vi "ZPL CheckSum Append.vi"(8 "error":errorcluster, 10 "Input Cmd":string, 11 "VISA":refnum<visa-resource-name>="COM1") -> (0 "error out":errorcluster, 2 "ChkSum Cmd":string, 3 "VISA out":refnum<visa-resource-name>)   [LabVIEW 2016]
doc: "This vi will add a checksum to any command string.\nThe format of the \"ChkSum Cmd\" output is:\n \"Command\" & \"Dollar Sign\" & \"Two Hex Digits\" & \"Carriage Return\"\n\nThe command is only formulated, it is not sent to the instrument."
panel:
  # "Add Checksum to \n  Command"
  # "Lambda ZPLUS \n  DC Power Supplies"
  # "Append \"$xx\" checksum to any\ncommand string if it is not already done"
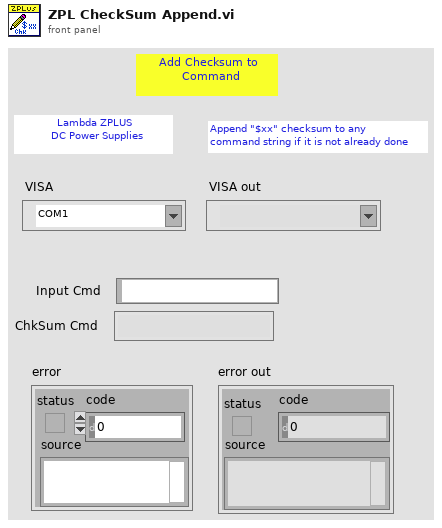
[diagram p1: front panel]
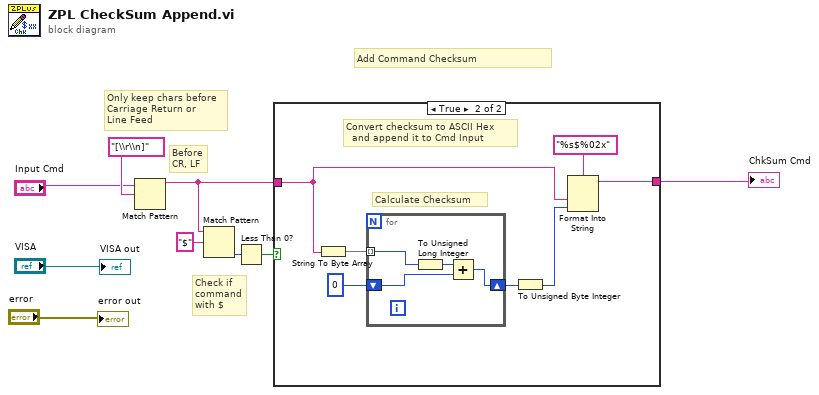
[diagram p0: block diagram]
diagram:
  # "Check if \ncommand\nwith $"
  # "Add Command Checksum"
  # "Before\nCR, LF"
  # "Only keep chars before\nCarriage Return or\nLine Feed"
  n1 = Match Pattern(string="Input Cmd", regular expression="[\\r\\n]") -> (before substring=w3:string)  [unwired: 1 in, 3 out]
  n2 = Match Pattern(string=w3, regular expression="$") -> (offset past match=w2:i32)  [unwired: 1 in, 3 out]
  n3 = Less Than 0?(x=w2) -> (x < 0?=w1:bool)
  n4 = case shown="True" w1 {
    tunnel: w3 -> [w10 w17]
    tunnel: [w10 w11] -> w5
    frame False {
      # "command\nwith $"
    }
    frame True {
      # "Convert checksum to ASCII Hex  \n  and append it to Cmd Input"
      # "Calculate Checksum"
      n5 = String To Byte Array(string=w17) -> (unsigned byte array=w16:u8[])
      n6 = for {
        tunnel: w16 -> [w21] mode=indexing
        shift-right: [w19] -> w14
        shift-left: u32 0 -> [w20]
        n7 = To Unsigned Long Integer(number=w21) -> (unsigned 32bit integer=w18:u32)
        n8 = Add(x=w18, y=w20) -> (x+y=w19:u32)
      }
      n9 = To Unsigned Byte Integer(number=w14) -> (unsigned 8bit integer=w12:u8)
      n10 = Format Into String(format string="%s$%02x" ("regular expression"), w17, w12) -> (resulting string=w11:string)  [unwired: 2 in, 1 out]
    }
  }
  "ChkSum Cmd" <- w5
  "error out" <- "error"
  "VISA out" <- "VISA"
